vi "HFRR ADV v01.vi"() -> ()   [LabVIEW 2025] (continued)
        n1285 = local write "Zoom Factore"(100.0 ("Zoom Factore")) -> ()
        n1286 = Strip Path(path=w1421) -> (name=w1424:string)  [unwired: 1 out]
        n1287 = Match Pattern(string=w1424, regular expression=w1422) -> (match substring=w1423:string)  [unwired: 1 in, 3 out]
        n1288 = Equal?(x=w1423, y=w1422) -> (x = y?=w1420:bool)
        n1289 = case shown="False" w1420 {
          frame False {
            n1290 = local write "Magnification :"("10x" ("Magnification :")) -> ()
          }
          frame True {
            n1291 = local write "Magnification :"("5x" ("Magnification :")) -> ()
          }
        }
      }
    }
    n1292 = case shown="True" w1115 {
      selector: w1115 -> [_ w1403]
      tunnel: w1107 -> [w1400 w1408]
      tunnel: [w1400 w1402] -> _
      frame False {
      }
      frame True {
        n1293 = Not(x=w1403) -> (.not. x?=w1401:bool)
        n1294 = local read "Zoom Factore"() -> (w1406:dbl)
        n1295 = local write "OUT"(w1401) -> ()
        n1296 = call "IMAGE ANALYSIS.vi"("Enum"=POST_ANALYSIS_ENUM."ZOOM OUT", "error in"=w1408) -> ("error out"=w1402:errorcluster)  [unwired: 8 in, 1 out]
        n1297 = Divide(x=w1406, y=1.2) -> (x/y=w1404:dbl)
        n1298 = local write "Zoom Factore"(w1404) -> ()
      }
    }
    n1299 = case shown="True" w1116 {
      selector: w1116 -> [_ w1412]
      tunnel: w1107 -> [w1409 w1417]
      tunnel: [w1409 w1410] -> _
      frame False {
      }
      frame True {
        n1300 = Not(x=w1412) -> (.not. x?=w1411:bool)
        n1301 = local read "Zoom Factore"() -> (w1415:dbl)
        n1302 = local write "In"(w1411) -> ()
        n1303 = call "IMAGE ANALYSIS.vi"("Enum"=POST_ANALYSIS_ENUM."ZOOM IN", "error in"=w1417) -> ("error out"=w1410:errorcluster)  [unwired: 8 in, 1 out]
        n1304 = Multiply(x=w1415, y=1.2) -> (x*y=w1413:dbl)
        n1305 = local write "Zoom Factore"(w1413) -> ()
      }
    }
    n1306 = case shown="True" w1112 {
      selector: w1112 -> [_ w1384]
      tunnel: w1107 -> [w1382 w1386]
      tunnel: [w1382 w1385] -> _
      frame False {
      }
      frame True {
        n1307 = Not(x=w1384) -> (.not. x?=w1383:bool)
        n1308 = local write "Clear ROI Tool"(w1383) -> ()
        n1309 = call "IMAGE ANALYSIS.vi"("Enum"=POST_ANALYSIS_ENUM."CLEAR ROI", "error in"=w1386) -> ("error out"=w1385:errorcluster)  [unwired: 8 in, 1 out]
      }
    }
    n1310 = case shown="True" w1114 {
      selector: w1114 -> [_ w1396]
      tunnel: w1107 -> [w1394 w1399]
      tunnel: [w1394 w1397] -> _
      frame False {
      }
      frame True {
        n1311 = Not(x=w1396) -> (.not. x?=w1395:bool)
        n1312 = local write "line tool"(w1395) -> ()
        n1313 = call "IMAGE ANALYSIS.vi"("Enum"=POST_ANALYSIS_ENUM."DRAW LINE", "error in"=w1399) -> ("error out"=w1397:errorcluster)  [unwired: 8 in, 1 out]
      }
    }
    n1314 = case shown="True" w1113 {
      selector: w1113 -> [_ w1390]
      tunnel: w1107 -> [w1388 w1392]
      tunnel: [w1388 w1391] -> _
      frame False {
      }
      frame True {
        n1315 = Not(x=w1390) -> (.not. x?=w1389:bool)
        n1316 = local write "Rectangle Tool"(w1389) -> ()
        n1317 = call "IMAGE ANALYSIS.vi"("Enum"=POST_ANALYSIS_ENUM."DRAW REC", "error in"=w1392) -> ("error out"=w1391:errorcluster)  [unwired: 8 in, 1 out]
      }
    }
    n1318 = local read "SCAR MEASURMENT"() -> (w1100:enum32{"Auto Scar", "Manual Scar"})
    n1319 = local read "Fit to Screen Tool"() -> (w1109:bool)
    n1320 = local read "Resize Tool"() -> (w1108:bool)
    n1321 = case shown="\"Manual Scar\", Default" w1100 {
      frame "Auto Scar" {
        n1322 = property on="Cap Live Image" class="Bool (strict)"("BoolText.Text"="Report" ("Boolean Text.Text")) -> ()  [unwired: 2 in, 2 out]
      }
      frame "Manual Scar", Default {
        n1323 = property on="Cap Live Image" class="Bool (strict)"("BoolText.Text"="Save Image" ("Boolean Text.Text")) -> ()  [unwired: 2 in, 2 out]
      }
    }
    n1324 = local read "ROI Color Tool"() -> (w1110:bool)
    n1325 = local read "Pan Tool"() -> (w1111:bool)
    n1326 = case shown="True" w1111 {
      selector: w1111 -> [_ w1378]
      tunnel: w1107 -> [w1376 w1380]
      tunnel: [w1376 w1379] -> _
      frame False {
      }
      frame True {
        n1327 = Not(x=w1378) -> (.not. x?=w1377:bool)
        n1328 = call "IMAGE ANALYSIS.vi"("Enum"=POST_ANALYSIS_ENUM."PAN", "error in"=w1380) -> ("error out"=w1379:errorcluster)  [unwired: 8 in, 1 out]
        n1329 = local write "Pan Tool"(w1377) -> ()
      }
    }
    n1330 = case shown="True" w1108 {
      selector: w1108 -> [_ w1362]
      tunnel: w1107 -> [w1357 w1359]
      tunnel: [w1357 w1358] -> _
      frame False {
      }
      frame True {
        n1331 = Not(x=w1362) -> (.not. x?=w1361:bool)
        n1332 = local write "Resize Tool"(w1361) -> ()
        n1333 = call "IMAGE ANALYSIS.vi"("Enum"=POST_ANALYSIS_ENUM."RESIZE MODE", "error in"=w1359) -> ("error out"=w1358:errorcluster)  [unwired: 8 in, 1 out]
      }
    }
    n1334 = case shown="True" w1109 {
      selector: w1109 -> [_ w1367]
      tunnel: [w1363 w1368] -> _
      tunnel: w1107 -> [w1363 w1366]
      frame False {
      }
      frame True {
        n1335 = Not(x=w1367) -> (.not. x?=w1365:bool)
        n1336 = local write "Zoom Factore"(100.0 ("Zoom Factore")) -> ()
        n1337 = local write "Fit to Screen Tool"(w1365) -> ()
        n1338 = call "IMAGE ANALYSIS.vi"("Enum"=POST_ANALYSIS_ENUM."FIT", "error in"=w1366) -> ("error out"=w1368:errorcluster)  [unwired: 8 in, 1 out]
      }
    }
    n1339 = case shown="True" w1110 {
      selector: w1110 -> [_ w1373]
      tunnel: [w1370 w1374] -> _
      tunnel: w1107 -> [w1370 w1371]
      frame False {
      }
      frame True {
        n1340 = Not(x=w1373) -> (.not. x?=w1372:bool)
        n1341 = local write "ROI Color Tool"(w1372) -> ()
        n1342 = call "IMAGE ANALYSIS.vi"("Enum"=POST_ANALYSIS_ENUM."SET ROI COLOR", "error in"=w1371) -> ("error out"=w1374:errorcluster)  [unwired: 8 in, 1 out]
      }
    }
    n1343 = local read "Quit"() -> (w1124:bool)
  }
  n1344 = while {
    stop <- w1469 stop-if-true
    n1345 = local read "Image Path"() -> (w1472:path)
    n1346 = local read "Print 3"() -> (w1475:bool)
    n1347 = Equal?(x=w1472, y=path "") -> (x = y?=w1471:bool)
    n1348 = Not(x=w1471) -> (.not. x?=w1470:bool)
    n1349 = property on="Print 3" class="Bool (strict)"("Visible"=w1470) -> ()  [unwired: 2 in, 2 out]
    n1350 = case shown="True" w1475 {
      frame False {
        n1351 = local write "Rd"(TRUE ("Boolean 7")) -> ()
      }
      frame True {
        n1352 = flat-sequence {
          tunnel: [w1515] -> w1483
          tunnel: [w1502] -> w1481
          tunnel: [w1512] -> w1477
          tunnel: w1483 -> [w1524]
          tunnel: [w1524] -> w1482
          tunnel: w1481 -> [w1523]
          tunnel: [w1523] -> w1480
          tunnel: [w1521] -> w1479
          tunnel: [w1520] -> w1478
          tunnel: w1477 -> [w1520]
          tunnel: w1482 -> [w1526]
          tunnel: w1480 -> [w1527]
          tunnel: w1479 -> [_]
          tunnel: w1478 -> [w1525]
          frame #0 {
            n1353 = case shown="True" "Rd" {
              frame False {
              }
              frame True {
                n1354 = while {
                  tunnel: "abcdefABCDEF" ("string 2") -> [w1494]
                  shift-right: [w1492] -> w1486
                  shift-left: "" -> [w1491]
                  i -> [w1501]
                  stop <- w1500 stop-if-true
                  n1355 = Random Number (0-1)() -> (number: 0 to 1=w1495:dbl)
                  n1356 = Multiply(x=w1495, y=62.0) -> (x*y=w1497:dbl)
                  n1357 = Decrement(x="Length 2") -> (x-1=w1490:i16)
                  n1358 = To Word Integer(number=w1497) -> (16bit integer=w1498:i16)
                  n1359 = String Subset(string=w1494, offset (0)=w1498, length (rest)=1 ("length (rest)")) -> (substring=w1493:string)
                  n1360 = Greater Or Equal?(x=w1501, y=w1490) -> (x >= y?=w1500:bool)
                  n1361 = Concatenate Strings(w1493, w1491) -> (w1492:string)
                }
                "String 10" <- w1486
                n1362 = local write "Rd"(FALSE ("Boolean 7")) -> ()
              }
            }
          }
          frame #1 {
            w1513 = "_resized.jpg" ("command line")
            (unwired) ".jpg -resize 320x240 " ("string")
            (unwired) "Choose an Image File" ("prompt")
            # "-resize 1798x425"
            n1363 = local read "Image Path"() -> (w1507:path)
            n1364 = Strip Path(path=w1507) -> (stripped path=w1502:path, name=w1503:string)
            n1365 = Match Pattern(string=w1503, regular expression=".jpg") -> (before substring=→"before substring 2":string, after substring=→"after substring":string)  [unwired: 1 in, 2 out]
            n1366 = Match Pattern(string=w1503, regular expression="\\") -> (before substring=w1509:string)  [unwired: 1 in, 3 out]
            n1367 = Match Pattern(string=w1509, regular expression=".jpg") -> (before substring=w1508:string)  [unwired: 1 in, 3 out]
            n1368 = Concatenate Strings("cmd /c convert " ("string"), w1508, ".jpg -resize 320x240  " ("command line"), w1508, w1513) -> (w1516:string)
            n1369 = call <vilib>:"System Exec.vi"("run minimized? (F)"=TRUE, "wait until completion? (T)"=TRUE, "working directory"=w1502, "command line"=w1516) -> ("error out"=w1515:errorcluster)  [unwired: 4 in, 3 out]
            "error out 2" <- w1515
            n1370 = Concatenate Strings(w1508, w1513) -> (w1512:string)
          }
          frame #2 {
            n1371 = Wait (ms)(milliseconds to wait=u32 2000 ("millisecond timer value")) -> (millisecond timer value=w1521:u32)
          }
          frame #3 {
            n1372 = case shown="No Error" w1526 {
              tunnel: w1527 -> [w1530 _]
              tunnel: w1525 -> [w1528 _]
              frame No Error {
                (unwired) ".jpg" ("string")
                n1373 = Path To String(path=w1530) -> (string=w1534:string)
                n1374 = Concatenate Strings(w1534, "\\" ("string"), w1528) -> (w1533:string)
                n1375 = String To Path(string=w1533) -> (path=w1532:path)
                n1376 = call <vilib>:"Read JPEG File.vi"("path to JPEG file"=w1532) -> ("image data"=w1536:T2)  [unwired: 8 in, 2 out]
                "image data" <- w1536
                n1377 = local write "Print 3"(FALSE ("Print 2")) -> ()
                n1378 = call <vilib>:"Draw Flattened Pixmap.vi"("image data"=w1536) -> ("new picture"=→"new picture":picture)  [unwired: 8 in]
              }
              frame Error {
              }
            }
          }
        }
      }
    }
    n1379 = Wait (ms)(milliseconds to wait=u32 20 ("millisecond timer value")) -> ()  [unwired: 1 out]
    n1380 = local read "Quit"() -> (w1469:bool)
  }
  n1381 = while {
    tunnel: w44 -> [_]
    tunnel: w30 -> [_]
    stop <- w1565 stop-if-true
    # "New Adv Logics"
    n1382 = local read "Main Tab"() -> (w1548:T4)
    n1383 = local read "Sign In"() -> (w1563:bool)
    n1384 = case shown="\"Advance\"" w1548 {
      frame "HOME", Default {
        n1385 = local read "LIVE FEED MIN TEMP"() -> (w1713:bool)
        n1386 = local write "LIVE FEED MAX TEMP"(TRUE ("LIVE FEED MAX TEMP")) -> ()
        n1387 = local read "CAMERA ROI MIN TEMP"() -> (w1711:bool)
        n1388 = case shown="True" w1713 {
          selector: w1713 -> [_ w1720]
          frame False {
          }
          frame True {
            n1389 = Not(x=w1720) -> (.not. x?=w1719:bool)
            n1390 = local write "LIVE FEED MIN TEMP"(w1719) -> ()
            n1391 = call "CAMERA LIVE FEED FGV.vi"("Enum - Menu"=CAMERA_LIVE_FEED_ENUM."CAMERA MINIMIZE") -> ()  [unwired: 9 in, 2 out]
          }
        }
        n1392 = case shown="True" w1711 {
          selector: w1711 -> [_ w1717]
          frame False {
          }
          frame True {
            n1393 = Not(x=w1717) -> (.not. x?=w1716:bool)
            n1394 = local write "CAMERA ROI MIN TEMP"(w1716) -> ()
            n1395 = call "IMAGE ANALYSIS.vi"("Enum"=POST_ANALYSIS_ENUM."MINIMIZE UI") -> ()  [unwired: 9 in, 2 out]
          }
        }
        n1396 = local write "CAMERA ROI MAX TEMP"(TRUE ("CAMERA ROI MAX TEMP")) -> ()
      }
      frame "Test Setup" {
        n1397 = local read "LIVE FEED MIN TEMP"() -> (w1723:bool)
        n1398 = local read "CAMERA ROI MIN TEMP"() -> (w1721:bool)
        n1399 = local write "LIVE FEED MAX TEMP"(TRUE ("LIVE FEED MAX TEMP")) -> ()
        n1400 = case shown="True" w1723 {
          selector: w1723 -> [_ w1730]
          frame False {
          }
          frame True {
            n1401 = Not(x=w1730) -> (.not. x?=w1729:bool)
            n1402 = local write "LIVE FEED MIN TEMP"(w1729) -> ()
            n1403 = call "CAMERA LIVE FEED FGV.vi"("Enum - Menu"=CAMERA_LIVE_FEED_ENUM."CAMERA MINIMIZE") -> ()  [unwired: 9 in, 2 out]
          }
        }
        n1404 = case shown="True" w1721 {
          selector: w1721 -> [_ w1727]
          frame False {
          }
          frame True {
            n1405 = Not(x=w1727) -> (.not. x?=w1726:bool)
            n1406 = local write "CAMERA ROI MIN TEMP"(w1726) -> ()
            n1407 = call "IMAGE ANALYSIS.vi"("Enum"=POST_ANALYSIS_ENUM."MINIMIZE UI") -> ()  [unwired: 9 in, 2 out]
          }
        }
        n1408 = local write "CAMERA ROI MAX TEMP"(TRUE ("CAMERA ROI MAX TEMP")) -> ()
      }
      frame "Acquire" {
        n1409 = local read "LIVE FEED MIN TEMP"() -> (w1733:bool)
        n1410 = local write "LIVE FEED MAX TEMP"(TRUE ("LIVE FEED MAX TEMP")) -> ()
        n1411 = local read "CAMERA ROI MIN TEMP"() -> (w1731:bool)
        n1412 = case shown="True" w1733 {
          selector: w1733 -> [_ w1740]
          frame False {
          }
          frame True {
            n1413 = Not(x=w1740) -> (.not. x?=w1739:bool)
            n1414 = local write "LIVE FEED MIN TEMP"(w1739) -> ()
            n1415 = call "CAMERA LIVE FEED FGV.vi"("Enum - Menu"=CAMERA_LIVE_FEED_ENUM."CAMERA MINIMIZE") -> ()  [unwired: 9 in, 2 out]
          }
        }
        n1416 = case shown="True" w1731 {
          selector: w1731 -> [_ w1737]
          frame False {
          }
          frame True {
            n1417 = Not(x=w1737) -> (.not. x?=w1736:bool)
            n1418 = local write "CAMERA ROI MIN TEMP"(w1736) -> ()
            n1419 = call "IMAGE ANALYSIS.vi"("Enum"=POST_ANALYSIS_ENUM."MINIMIZE UI") -> ()  [unwired: 9 in, 2 out]
          }
        }
        n1420 = local write "CAMERA ROI MAX TEMP"(TRUE ("CAMERA ROI MAX TEMP")) -> ()
      }
      frame "Adv Scar" {
        n1421 = local read "CAMERA ROI MIN TEMP"() -> (w1741:bool)
        n1422 = case shown="True" "LIVE FEED MAX TEMP" {
          selector: "LIVE FEED MAX TEMP" -> [_ w1762]
          frame False {
          }
          frame True {
            n1423 = Not(x=w1762) -> (.not. x?=w1761:bool)
            n1424 = local write "LIVE FEED MAX TEMP"(w1761) -> ()
            n1425 = call "CAMERA LIVE FEED FGV.vi"("Enum - Menu"=CAMERA_LIVE_FEED_ENUM."CAMERA RESTORE") -> ("error out"=w1752:errorcluster)  [unwired: 9 in, 1 out]
            n1426 = Type Cast(type=30, x=0) -> (*(type *) &x=w1756:i32)
            n1427 = Add(x=w1756, y=48) -> (x+y=w1757:i32)
            n1428 = call "CAMERA LIVE FEED FGV.vi"("Enum - Menu"=CAMERA_LIVE_FEED_ENUM."CAMERA MODE SET", "error in (no error)"=w1752, "CAMERA MODE"=w1757) -> ("error out"=w1749:errorcluster)  [unwired: 7 in, 1 out]
            n1429 = call "CAMERA LIVE FEED FGV.vi"("Enum - Menu"=CAMERA_LIVE_FEED_ENUM."CAMERA GRAY", "error in (no error)"=w1749) -> ("error out"=w1748:errorcluster)  [unwired: 8 in, 1 out]
            n1430 = call "LIST FILE NAMES.vi"("error in (no error)"=w1748) -> ("error out"=w1758:errorcluster, "filenames"=w1759:string[])  [unwired: 9 in]
            n1431 = property on="FILE 3" class="CmbBox"(error in=w1758, "Strings[]"=w1759) -> ()  [unwired: 1 in, 2 out]
          }
        }
        n1432 = case shown="True" w1741 {
          selector: w1741 -> [_ w1747]
          frame False {
          }
          frame True {
            n1433 = Not(x=w1747) -> (.not. x?=w1746:bool)
            n1434 = local write "CAMERA ROI MIN TEMP"(w1746) -> ()
            n1435 = call "IMAGE ANALYSIS.vi"("Enum"=POST_ANALYSIS_ENUM."MINIMIZE UI") -> ()  [unwired: 9 in, 2 out]
          }
        }
        n1436 = local write "CAMERA ROI MAX TEMP"(TRUE ("CAMERA ROI MAX TEMP")) -> ()
        "LIVE FEED MIN TEMP" <- TRUE ("LIVE FEED MIN TEMP")
      }
      frame "Adv Scar Report" {
        n1437 = local read "CAMERA ROI MAX TEMP"() -> (w1763:bool)
        n1438 = local read "LIVE FEED MIN TEMP"() -> (w1765:bool)
        n1439 = local write "LIVE FEED MAX TEMP"(TRUE ("LIVE FEED MAX TEMP")) -> ()
        n1440 = case shown="True" w1765 {
          selector: w1765 -> [_ w1774]
          frame False {
          }
          frame True {
            n1441 = Not(x=w1774) -> (.not. x?=w1773:bool)
            n1442 = local write "LIVE FEED MIN TEMP"(w1773) -> ()
            n1443 = call "CAMERA LIVE FEED FGV.vi"("Enum - Menu"=CAMERA_LIVE_FEED_ENUM."CAMERA MINIMIZE") -> ()  [unwired: 9 in, 2 out]
          }
        }
        n1444 = case shown="True" w1763 {
          selector: w1763 -> [_ w1771]
          frame False {
          }
          frame True {
            n1445 = Not(x=w1771) -> (.not. x?=w1769:bool)
            n1446 = local write "CAMERA ROI MAX TEMP"(w1769) -> ()
            n1447 = call "IMAGE ANALYSIS.vi"("Enum"=POST_ANALYSIS_ENUM."SHOW UI") -> ("error out"=w1768:errorcluster)  [unwired: 9 in, 1 out]
            n1448 = call "LIST FILE NAMES.vi"("error in (no error)"=w1768) -> ("filenames"=w1767:string[])  [unwired: 9 in, 1 out]
            n1449 = property on="Test File List :" class="CmbBox"("Strings[]"=w1767) -> ()  [unwired: 2 in, 2 out]
          }
        }
        n1450 = local write "CAMERA ROI MIN TEMP"(TRUE ("CAMERA ROI MIN TEMP")) -> ()
      }
      frame "Compare Files" {
        n1451 = local read "LIVE FEED MIN TEMP"() -> (w1777:bool)
        n1452 = local write "LIVE FEED MAX TEMP"(TRUE ("LIVE FEED MAX TEMP")) -> ()
        n1453 = local read "CAMERA ROI MIN TEMP"() -> (w1775:bool)
        n1454 = case shown="True" w1777 {
          selector: w1777 -> [_ w1784]
          frame False {
          }
          frame True {
            n1455 = Not(x=w1784) -> (.not. x?=w1783:bool)
            n1456 = local write "LIVE FEED MIN TEMP"(w1783) -> ()
            n1457 = call "CAMERA LIVE FEED FGV.vi"("Enum - Menu"=CAMERA_LIVE_FEED_ENUM."CAMERA MINIMIZE") -> ()  [unwired: 9 in, 2 out]
          }
        }
        n1458 = case shown="True" w1775 {
          selector: w1775 -> [_ w1781]
          frame False {
          }
          frame True {
            n1459 = Not(x=w1781) -> (.not. x?=w1780:bool)
            n1460 = local write "CAMERA ROI MIN TEMP"(w1780) -> ()
            n1461 = call "IMAGE ANALYSIS.vi"("Enum"=POST_ANALYSIS_ENUM."MINIMIZE UI") -> ()  [unwired: 9 in, 2 out]
          }
        }
        n1462 = local write "CAMERA ROI MAX TEMP"(TRUE ("CAMERA ROI MAX TEMP")) -> ()
      }
      frame "About" {
        n1463 = local read "LIVE FEED MIN TEMP"() -> (w1787:bool)
        n1464 = local write "LIVE FEED MAX TEMP"(TRUE ("LIVE FEED MAX TEMP")) -> ()
        n1465 = local read "CAMERA ROI MIN TEMP"() -> (w1786:bool)
        n1466 = case shown="True" w1787 {
          selector: w1787 -> [_ w1794]
          frame False {
          }
          frame True {
            n1467 = Not(x=w1794) -> (.not. x?=w1793:bool)
            n1468 = local write "LIVE FEED MIN TEMP"(w1793) -> ()
            n1469 = call "CAMERA LIVE FEED FGV.vi"("Enum - Menu"=CAMERA_LIVE_FEED_ENUM."CAMERA MINIMIZE") -> ()  [unwired: 9 in, 2 out]
          }
        }
        n1470 = case shown="True" w1786 {
          selector: w1786 -> [_ w1791]
          frame False {
          }
          frame True {
            n1471 = Not(x=w1791) -> (.not. x?=w1790:bool)
            n1472 = local write "CAMERA ROI MIN TEMP"(w1790) -> ()
            n1473 = call "IMAGE ANALYSIS.vi"("Enum"=POST_ANALYSIS_ENUM."MINIMIZE UI") -> ()  [unwired: 9 in, 2 out]
          }
        }
        n1474 = local write "CAMERA ROI MAX TEMP"(TRUE ("CAMERA ROI MIN TEMP")) -> ()
      }
      frame "Advance" {
        n1475 = local read "LIVE FEED MIN TEMP"() -> (w1797:bool)
        n1476 = local write "LIVE FEED MAX TEMP"(TRUE ("LIVE FEED MAX TEMP")) -> ()
        n1477 = local read "CAMERA ROI MIN TEMP"() -> (w1795:bool)
        n1478 = case shown="True" w1797 {
          selector: w1797 -> [_ w1804]
          frame False {
          }
          frame True {
            n1479 = Not(x=w1804) -> (.not. x?=w1803:bool)
            n1480 = local write "LIVE FEED MIN TEMP"(w1803) -> ()
            n1481 = call "CAMERA LIVE FEED FGV.vi"("Enum - Menu"=CAMERA_LIVE_FEED_ENUM."CAMERA MINIMIZE") -> ()  [unwired: 9 in, 2 out]
          }
        }
        n1482 = local write "CAMERA ROI MAX TEMP"(TRUE ("CAMERA ROI MAX TEMP")) -> ()
        n1483 = case shown="True" w1795 {
          selector: w1795 -> [_ w1801]
          frame False {
          }
          frame True {
            n1484 = Not(x=w1801) -> (.not. x?=w1800:bool)
            n1485 = local write "CAMERA ROI MIN TEMP"(w1800) -> ()
            n1486 = call "IMAGE ANALYSIS.vi"("Enum"=POST_ANALYSIS_ENUM."MINIMIZE UI") -> ()  [unwired: 9 in, 2 out]
          }
        }
      }
      frame "Mooha" {
        n1487 = local read "LIVE FEED MIN TEMP"() -> (w1807:bool)
        n1488 = local write "LIVE FEED MAX TEMP"(TRUE ("LIVE FEED MAX TEMP")) -> ()
        n1489 = local read "CAMERA ROI MIN TEMP"() -> (w1805:bool)
        n1490 = case shown="True" w1807 {
          selector: w1807 -> [_ w1814]
          frame False {
          }
          frame True {
            n1491 = Not(x=w1814) -> (.not. x?=w1813:bool)
            n1492 = local write "LIVE FEED MIN TEMP"(w1813) -> ()
            n1493 = call "CAMERA LIVE FEED FGV.vi"("Enum - Menu"=CAMERA_LIVE_FEED_ENUM."CAMERA MINIMIZE") -> ()  [unwired: 9 in, 2 out]
          }
        }
        n1494 = local write "CAMERA ROI MAX TEMP"(TRUE ("CAMERA ROI MAX TEMP")) -> ()
        n1495 = case shown="True" w1805 {
          selector: w1805 -> [_ w1811]
          frame False {
          }
          frame True {
            n1496 = Not(x=w1811) -> (.not. x?=w1810:bool)
            n1497 = local write "CAMERA ROI MIN TEMP"(w1810) -> ()
            n1498 = call "IMAGE ANALYSIS.vi"("Enum"=POST_ANALYSIS_ENUM."MINIMIZE UI") -> ()  [unwired: 9 in, 2 out]
          }
        }
      }
    }
    n1499 = property on="DEMO" class="Bool (strict)"() -> ("Value"=w1537:bool)  [unwired: 2 in, 2 out]
    n1500 = local read "Auto Start Test"() -> (w1540:bool)
    n1501 = case shown="False" w1537 {
      frame False {
        n1502 = local read "Main Tab"() -> (w1566:T4)
        n1503 = case shown="\"HOME\"" w1566 {
          frame "HOME" {
            n1504 = local write "main tab sub"(enum32{"Page 1", "Page 2"}."Page 1" ("main tab sub")) -> ()
          }
          frame Default {
            n1505 = local write "main tab sub"(enum32{"Page 1", "Page 2"}."Page 2" ("main tab sub")) -> ()
          }
        }
      }
      frame True {
      }
    }
    n1506 = case shown="True" "sign in temp" {
      frame False {
      }
      frame True {
        w1651 = 1 ("y")
        n1507 = local read "USERNAME"() -> (w1657:string)
        n1508 = local read "USER ID"() -> (w1654:string)
        n1509 = call <vilib>:"Trim Whitespace.vi"("string"=w1657) -> ("trimmed string"=w1656:string)  [unwired: 1 in]
        n1510 = call <vilib>:"Trim Whitespace.vi"("string"=w1654) -> ("trimmed string"=w1655:string)  [unwired: 1 in]
        n1511 = String Length(string=w1656) -> (length=w1653:i32)
        n1512 = String Length(string=w1655) -> (length=w1652:i32)
        n1513 = Greater?(x=w1653, y=w1651) -> (0:w1650:bool)
        n1514 = Greater?(x=w1652, y=w1651) -> (0:w1649:bool)
        n1515 = And(x=w1650, y=w1649) -> (x .and. y?=w1648:bool)
        n1516 = case shown="True" w1648 {
          frame False {
            n1517 = property on="Sign In" class="Bool (strict)"("DisabledEnum"=T20."Disabled" ("Disabled")) -> ()  [unwired: 2 in, 2 out]
          }
          frame True {
            n1518 = property on="Sign In" class="Bool (strict)"("DisabledEnum"=T20."Enabled" ("Disabled")) -> ()  [unwired: 2 in, 2 out]
          }
        }
      }
    }
    n1519 = local read "Air Temperature"() -> (w1556:bool)
    n1520 = property on="DEMO" class="Bool (strict)"() -> ("Value"=w1538:bool)  [unwired: 2 in, 2 out]
    n1521 = local read "Coefficient Of Friction"() -> (w1557:bool)
    n1522 = case shown="False" w1540 {
      frame False {
        n1523 = local read "Auto stop temp"() -> (w1645:bool)
        n1524 = case shown="True" w1645 {
          frame False {
          }
          frame True {
            n1525 = local write "Auto Start Temp"(FALSE ("Auto Start Temp")) -> ()
          }
        }
      }
      frame True {
        "Auto stop temp" <- TRUE ("Auto stop temp")
      }
    }
    n1526 = local read "Humidity 3"() -> (w1555:bool)
    n1527 = case shown="True" w1563 {
      selector: w1563 -> [_ w1920]
      frame False {
      }
      frame True {
        n1528 = Not(x=w1920) -> (.not. x?=w1919:bool)
        n1529 = local write "Sign In"(w1919) -> ()
        n1530 = local write "Main Dashboard Buttons"(T26."Test Setup" ("Main Dashboard Buttons")) -> ()
      }
    }
    n1531 = case shown="\"Numeric Display\", Default" "Num/Graph" {
      frame "Numeric Display", Default {
        n1532 = property on="Single/Multiple" class="RadioBtnsControl (strict)"("Visible"=FALSE) -> ()  [unwired: 2 in, 2 out]
        n1533 = property on="Single - Graph" class="Ring (strict)"("Visible"=FALSE) -> ()  [unwired: 2 in, 2 out]
        n1534 = local write "Main Tab Display"(T6."Dashboard 1" ("Main Tab Display")) -> ()
      }
      frame "Graph Display" {
        n1535 = property on="Single/Multiple" class="RadioBtnsControl (strict)"("Visible"=TRUE) -> ()  [unwired: 2 in, 2 out]
        n1536 = case shown="\"Multiple\"" "Single/Multiple" {
          frame "Single ", Default {
            n1537 = property on="Single - Graph" class="Ring (strict)"("Visible"=TRUE) -> ()  [unwired: 2 in, 2 out]
            n1538 = local write "Main Tab Display"(T6."Dashboard 3" ("Main Tab Display")) -> ()
          }
          frame "Multiple" {
            n1539 = property on="Single - Graph" class="Ring (strict)"("Visible"=FALSE) -> ()  [unwired: 2 in, 2 out]
            n1540 = local write "Main Tab Display"(T6."Dashboard 2" ("Main Tab Display")) -> ()
          }
        }
      }
    }
    n1541 = local read "Stroke"() -> (w1554:bool)
    n1542 = local read "USERNAME"() -> (w1559:string)
    n1543 = case shown="False" w1538 {
      frame False {
        n1544 = case shown="\"Calibration\"" "Main Dashboard Buttons" {
          tunnel: [T4."HOME" ("Main Tab") T4."Test Setup" ("Main Tab") T4."Acquire" ("Main Tab") T4."Adv Scar" ("Main Tab") T4."Adv Scar Report" ("Main Tab") T4."Compare Files" ("Main Tab") T4."Calibration" ("Main Tab") T4."About" ("Main Tab") T4."Advance" ("Main Tab")] -> w1569
          frame "Home", Default {
          }
          frame "Test Setup" {
          }
          frame "Dashboard" {
          }
          frame "Imaging" {
          }
          frame "Report" {
          }
          frame "Analysis" {
          }
          frame "Calibration" {
          }
          frame "About" {
          }
          frame "Advance" {
          }
        }
        n1545 = local write "Main Tab"(w1569) -> ()
      }
      frame True {
      }
    }
    n1546 = case shown="True" w1557 {
      selector: w1557 -> [_ w1854]
      frame False {
      }
      frame True {
        n1547 = Not(x=w1854) -> (.not. x?=w1853:bool)
        n1548 = local write "Coefficient Of Friction"(w1853) -> ()
        n1549 = local write "Tab Control 2"(T8."Coefficient Of Friction" ("Tab Control 2")) -> ()
      }
    }
    n1550 = case shown="True" w1556 {
      selector: w1556 -> [_ w1851]
      frame False {
      }
      frame True {
        n1551 = Not(x=w1851) -> (.not. x?=w1849:bool)
        n1552 = local write "Air Temperature"(w1849) -> ()
        n1553 = local write "Tab Control 2"(T8."Air Temperature" ("Tab Control 2")) -> ()
      }
    }
    n1554 = case shown="True" w1554 {
      selector: w1554 -> [_ w1845]
      frame False {
      }
      frame True {
        n1555 = Not(x=w1845) -> (.not. x?=w1843:bool)
        n1556 = local write "Stroke"(w1843) -> ()
        n1557 = local write "Tab Control 2"(T8."Stroke" ("Tab Control 2")) -> ()
      }
    }
    n1558 = local write "tested by"(w1559) -> ()
    n1559 = case shown="True" w1555 {
      selector: w1555 -> [_ w1848]
      frame False {
      }
      frame True {
        n1560 = Not(x=w1848) -> (.not. x?=w1846:bool)
        n1561 = local write "Humidity 3"(w1846) -> ()
        n1562 = local write "Tab Control 2"(T8."Humidity" ("Tab Control 2")) -> ()
      }
    }
    n1563 = Wait (ms)(milliseconds to wait=u32 100) -> ()  [unwired: 1 out]
    n1564 = local read "Main Tab Display"() -> (w1558:T6)
    n1565 = case shown="\"Dashboard 3\"" w1558 {
      frame "Dashboard 1", Default {
        n1566 = property on="Reset Graph" class="Bool (strict)"("Visible"=FALSE) -> ()  [unwired: 2 in, 2 out]
      }
      frame "Dashboard 2" {
        n1567 = property on="Reset Graph" class="Bool (strict)"("Visible"=TRUE) -> ()  [unwired: 2 in, 2 out]
      }
      frame "Dashboard 3" {
        n1568 = property on="Reset Graph" class="Bool (strict)"("Visible"=TRUE) -> ()  [unwired: 2 in, 2 out]
      }
    }
    n1569 = local read "SCAR MEASURMENT"() -> (w1546:enum32{"Auto Scar", "Manual Scar"})
    n1570 = local read "Humidity"() -> (w1560:bool)
    n1571 = local read "Cap Live Image"() -> (w1543:bool)
    n1572 = local read "Sample Temperature"() -> (w1553:bool)
    n1573 = local read "Air Temp vs Humidity"() -> (w1551:bool)
    n1574 = local read "Frequency"() -> (w1552:bool)
    n1575 = case shown="False" w1560 {
      frame False {
        n1576 = local write "Humidity On Command"(TRUE ("Humidity On Command")) -> ()
        n1577 = case shown="True" "Humidity Off Command" {
          selector: "Humidity Off Command" -> [_ w1861]
          frame False {
          }
          frame True {
            n1578 = stacked-sequence {
              frame #0 {
                n1579 = local read "WriteHumidity"() -> (w1863:string[])
                n1580 = Insert Into Array(array=w1863, new element="R;1" ("new element/subarray")) -> (w1862:string[])  [unwired: 1 in]
                n1581 = local write "WriteHumidity"(w1862) -> ()
              }
              frame #1 {
                n1582 = Wait (ms)(milliseconds to wait=u32 500) -> ()  [unwired: 1 out]
              }
              frame #2 {
                n1583 = local read "WriteHumidity"() -> (w1867:string[])
                n1584 = local read "EVENT LOG"() -> (w1871:string)
                n1585 = call "Event Log.vi"("Content"="Humidity Control Off" ("string"), "EVENT LOG"=w1871) -> ("EVENT LOG"=w1872:string)  [unwired: 8 in, 1 out]
                n1586 = local write "EVENT LOG"(w1872) -> ()
                n1587 = Insert Into Array(array=w1867, new element="R;1" ("new element/subarray")) -> (w1868:string[])  [unwired: 1 in]
                n1588 = local write "WriteHumidity"(w1868) -> ()
                n1589 = local write "Humidity 2"(TRUE ("Humidity")) -> ()
              }
            }
            n1590 = Not(x=w1861) -> (.not. x?=w1860:bool)
            n1591 = local write "Humidity Off Command"(w1860) -> ()
          }
        }
      }
      frame True {
        n1592 = local write "Humidity Off Command"(TRUE ("Humidity Off Command")) -> ()
        n1593 = case shown="False" "Humidity On Command" {
          selector: "Humidity On Command" -> [_ w1876]
          frame False {
          }
          frame True {
            n1594 = stacked-sequence {
              frame #0 {
                n1595 = local read "Set Rh"() -> (w1882:dbl)
                n1596 = local read "WriteHumidity"() -> (w1878:string[])
                n1597 = Number To Fractional String(number=w1882, precision (6)=i16 2) -> (F-format string=w1883:string)  [unwired: 2 in]
                n1598 = Concatenate Strings("M;" ("new element/subarray"), w1883) -> (w1881:string)
                n1599 = Insert Into Array(array=w1878, new element=w1881) -> (w1877:string[])  [unwired: 1 in]
                n1600 = local write "WriteHumidity"(w1877) -> ()
              }
              frame #1 {
                n1601 = Wait (ms)(milliseconds to wait=u32 500) -> ()  [unwired: 1 out]
              }
              frame #2 {
                n1602 = local read "WriteHumidity"() -> (w1886:string[])
                n1603 = local read "Set Rh"() -> (w1890:dbl)
                n1604 = Number To Fractional String(number=w1890, precision (6)=i16 2) -> (F-format string=w1891:string)  [unwired: 2 in]
                n1605 = Concatenate Strings("M;" ("new element/subarray"), w1891) -> (w1889:string)
                n1606 = Insert Into Array(array=w1886, new element=w1889) -> (w1885:string[])  [unwired: 1 in]
                n1607 = local write "WriteHumidity"(w1885) -> ()
              }
              frame #3 {
                n1608 = Wait (ms)(milliseconds to wait=u32 500) -> ()  [unwired: 1 out]
              }
              frame #4 {
                (unwired) "% RH" ("string")
                (unwired) i16 2 ("precision (6)")
                (unwired) "M;" ("new element/subarray")
                n1609 = local read "Set Rh"() -> (w1900:dbl)
                n1610 = local read "WriteHumidity"() -> (w1893:string[])
                n1611 = Number To Fractional String(number=w1900, precision (6)=i16 2) -> (F-format string=w1897:string)  [unwired: 2 in]
                n1612 = Concatenate Strings("M;" ("new element/subarray"), w1897) -> (w1901:string)
                n1613 = Concatenate Strings("Humidity Set to : " ("string"), w1897, "% RH" ("string")) -> (w1895:string)
                n1614 = Insert Into Array(array=w1893, new element=w1901) -> (w1894:string[])  [unwired: 1 in]
                n1615 = disable-structure shown="Enabled" {
                  frame Enabled {
                    n1616 = local read "EVENT LOG"() -> (w1904:string)
                    n1617 = call "Event Log.vi"("Content"="Humidity Control On", "EVENT LOG"=w1904) -> ("EVENT LOG"=w1905:string)  [unwired: 8 in, 1 out]
                    n1618 = local write "EVENT LOG"(w1905) -> ()
                  }
                  frame Disabled {
                  }
                }
                n1619 = disable-structure shown="Enabled" {
                  disable-tunnel: w1895 -> [_ _]
                  frame Enabled {
                    n1620 = local read "EVENT LOG"() -> (w1907:string)
                    n1621 = call "Event Log.vi"("Content"="Humidity Control On", "EVENT LOG"=w1907) -> ("EVENT LOG"=w1908:string)  [unwired: 8 in, 1 out]
                    n1622 = local write "EVENT LOG"(w1908) -> ()
                  }
                  frame Disabled {
                  }
                }
                n1623 = local write "WriteHumidity"(w1894) -> ()
              }
            }
            n1624 = Not(x=w1876) -> (.not. x?=w1875:bool)
            n1625 = local write "Humidity On Command"(w1875) -> ()
          }
        }
      }
    }
    n1626 = Equal?(x=w1546, y=enum32{"Auto Scar", "Manual Scar"}."Auto Scar" ("SCAR MEASURMENT")) -> (x = y?=w1542:bool)
    n1627 = local read "TEST STANDARD"() -> (w1549:T5)
    n1628 = And(x=w1543, y=w1542) -> (x .and. y?=w1544:bool)
    n1629 = case shown="True" w1544 {
      selector: w1544 -> [_ w1660]
      tunnel: errorcluster {"status"=FALSE, "code"=0, "source"=""} ("error in (no error) 3") -> [_ w1661]
      frame False {
      }
      frame True {
        n1630 = stacked-sequence {
          tunnel: w1661 -> [_ _ _ _ _ _ _ w1709]
          tunnel: w1660 -> [_ _ _ _ _ w1690 _ _]
          frame #0 {
            n1631 = call "CAMERA LIVE FEED FGV.vi"("Enum - Menu"=CAMERA_LIVE_FEED_ENUM."CAMERA MINIMIZE") -> ()  [unwired: 9 in, 2 out]
          }
          frame #1 {
            n1632 = property on="Auto Scar Check  2" class="Clust (strict)"("Visible"=TRUE) -> ()  [unwired: 2 in, 2 out]
          }
          frame #2 {
            n1633 = String To Path(string="C:\\LAB-IQ\\Image Calibrate v01.dcf") -> (path=w1666:path)
            n1634 = Open/Create/Replace File ("Open File")(file path (use dialog)=w1666) -> (refnum out=w1667:refnum<file>)  [unwired: 5 in, 2 out]
            n1635 = for {
              N: 4 -> [_]
              tunnel: w1667 -> [w1673]
              i -> [w1669]
              n1636 = Read from Text File ("Read File")(file (use dialog)=w1673) -> (text=w1674:string)  [unwired: 3 in, 3 out]
              n1637 = String Subset(string=w1674, offset (0)=6, length (rest)=10 ("length (rest)")) -> (substring=w1670:string)
              n1638 = Fract/Exp String To Number(string=w1670) -> (number=w1668:dbl)  [unwired: 3 in, 1 out]
              n1639 = case shown="0" w1669 {
                tunnel: w1668 -> [w1675 w1676 _ w1677 _]
                frame 0 {
                  "5x Gain" <- w1675
                }
                frame 1 {
                  "10x Gain" <- w1676
                }
                frame 2 {
                }
                frame 3 {
                  "100x gain" <- w1677
                }
                frame 4, Default {
                }
              }
            }
          }
          frame #3 {
            n1640 = local read "FILE 3"() -> (w1683:string)
            n1641 = call <vilib>:"Trim Whitespace.vi"("string"="C:\\LAB-IQ\\images\\") -> ("trimmed string"=w1685:string)  [unwired: 1 in]
            n1642 = String To Path(string=w1685) -> (path=w1684:path)
            n1643 = Concatenate Strings(w1683, ".png" ("string")) -> (w1682:string)
            n1644 = Build Path(base path=w1684, name or relative path=w1682) -> (appended path=w1680:path)
            "Image path" <- w1680
            n1645 = Path To String(path=w1680) -> (string=w1679:string)
            n1646 = call "CAMERA LIVE FEED FGV.vi"("Enum - Menu"=CAMERA_LIVE_FEED_ENUM."CAMERA SAVE", "Image Path"=w1679) -> ()  [unwired: 8 in, 2 out]
          }
          frame #4 {
            n1647 = One Button Dialog(message="Image saved successfully") -> ()  [unwired: 1 in, 1 out]
          }
          frame #5 {
            n1648 = local read "TEST STANDARD"() -> (w1689:T5)
            n1649 = local read "Magnification len live scar"() -> (w1701:string)
            n1650 = Not(x=w1690) -> (.not. x?=w1691:bool)
            n1651 = local write "Cap Live Image"(w1691) -> ()
            n1652 = case shown="\"ISO 12156\"" w1689 {
              tunnel: ["ASTM D6079" "ISO 12156"] -> w1688
              frame "ASTM D6079", Default {
              }
              frame "ISO 12156" {
              }
            }
            n1653 = case shown="\"5x\", Default" w1701 {
              tunnel: [w1704 w1705] -> w1700
              frame "5x", Default {
                n1654 = local read "5x Gain"() -> (w1704:dbl)
              }
              frame "10x" {
                # "5x"
                n1655 = local read "10x Gain"() -> (w1705:dbl)
              }
            }
            n1656 = local read "Image path"() -> (w1699:path)
            n1657 = local read "FILE 3"() -> (w1692:string)
            n1658 = call "EDGE DETCTION.vi"("GAIN VALUE"=w1700, "Image Path"=w1699) -> ("error out"=w1698:errorcluster, "return value"=w1697:cluster{string, string, dbl, dbl, dbl})  [unwired: 8 in]
            n1659 = Bundle By Name(cluster=T27 {"File Name"="", "Test Method"="", "Operator"="", "Fuel Description"="", "Date and time"=""} ("Main Ref"), "File Name"=w1692, "Test Method"=w1688) -> (w1693:T27)
            n1660 = call "duf file read.vi"("error in (no error)"=w1698, "Main Ref"=w1693) -> ("error out"=w1696:errorcluster, "Main Ref 2"=w1694:T27)  [unwired: 8 in]
            n1661 = call "EDGE DETECTION REPORT.vi"("error in (no error)"=w1696, "return value 2"=w1697, "Main Ref"=w1694) -> ()  [unwired: 8 in, 1 out]
          }
          frame #6 {
            n1662 = property on="Auto Scar Check  2" class="Clust (strict)"("Visible"=FALSE) -> ()  [unwired: 2 in, 2 out]
          }
          frame #7 {
            n1663 = call "CAMERA LIVE FEED FGV.vi"("Enum - Menu"=CAMERA_LIVE_FEED_ENUM."CAMERA MINIMIZE", "error in (no error)"=w1709) -> ()  [unwired: 8 in, 2 out]
            n1664 = local write "Main Dashboard Buttons"(T1."Home" ("Main Dashboard Buttons")) -> ()
            n1665 = local write "Main Tab"(T4."HOME" ("Main Tab")) -> ()
          }
        }
      }
    }
    n1666 = local read "Heater Button"() -> (w1550:bool)
    n1667 = case shown="True" w1552 {
      selector: w1552 -> [_ w1839]
      frame False {
      }
      frame True {
        n1668 = Not(x=w1839) -> (.not. x?=w1837:bool)
        n1669 = local write "Frequency"(w1837) -> ()
        n1670 = local write "Tab Control 2"(T8."Frequency" ("Tab Control 2")) -> ()
      }
    }
    n1671 = case shown="True" w1551 {
      selector: w1551 -> [_ w1836]
      frame False {
      }
      frame True {
        n1672 = Not(x=w1836) -> (.not. x?=w1834:bool)
        n1673 = local write "Air Temp vs Humidity"(w1834) -> ()
        n1674 = local write "Tab Control 2"(T8."Air Temp vs Rh" ("Tab Control 2")) -> ()
      }
    }
    n1675 = case shown="True" w1553 {
      selector: w1553 -> [_ w1842]
      frame False {
      }
      frame True {
        n1676 = Not(x=w1842) -> (.not. x?=w1840:bool)
        n1677 = local write "Sample Temperature"(w1840) -> ()
        n1678 = local write "Tab Control 2"(T8."Sample Temperature" ("Tab Control 2")) -> ()
      }
    }
    n1679 = case shown="\"Custom\"" w1549 {
      frame "ASTM D6079", Default {
        w1815 = "ASTM D6079 TEST CONDITIONS" ("Standard 2")
        n1680 = local write "Standard 2"(w1815) -> ()
        n1681 = local write "Standard"(w1815) -> ()
      }
      frame "ISO 12156" {
        w1816 = "ISO 12156 TEST CONDITIONS" ("Standard 2")
        n1682 = local write "Standard 2"(w1816) -> ()
        n1683 = local write "Standard"(w1816) -> ()
      }
      frame "CEC F-096-A-06" {
        w1817 = "CEC F-096-A-06 TEST CONDITIONS" ("Standard 2")
        n1684 = local write "Standard 2"(w1817) -> ()
        n1685 = local write "Standard"(w1817) -> ()
      }
      frame "Custom" {
        w1818 = "CUSTOM TEST CONDITIONS" ("Standard 2")
        n1686 = local write "Standard 2"(w1818) -> ()
        n1687 = local write "Standard"(w1818) -> ()
      }
    }
    n1688 = case shown="True" w1550 {
      frame False {
        n1689 = local write "Temperature On Command"(TRUE ("Temperature On Command")) -> ()
        n1690 = case shown="True" "Temperature Off Command" {
          selector: "Temperature Off Command" -> [_ w1822]
          frame False {
          }
          frame True {
            n1691 = Not(x=w1822) -> (.not. x?=w1821:bool)
            n1692 = local read "EVENT LOG"() -> (w1825:string)
            n1693 = local write "Temperature Off Command"(w1821) -> ()
            n1694 = call "Event Log.vi"("Content"="Heater Off", "EVENT LOG"=w1825) -> ("EVENT LOG"=w1824:string)  [unwired: 8 in, 1 out]
            n1695 = local write "EVENT LOG"(w1824) -> ()
          }
        }
      }
      frame True {
        n1696 = local write "Temperature Off Command"(TRUE ("Temperature Off Command")) -> ()
        n1697 = case shown="True" "Temperature On Command" {
          selector: "Temperature On Command" -> [_ w1829]
          frame False {
          }
          frame True {
            n1698 = Not(x=w1829) -> (.not. x?=w1828:bool)
            n1699 = local write "Temperature On Command"(w1828) -> ()
            n1700 = disable-structure shown="Enabled" {
              disable-tunnel: "Heater On" -> [w1831 _]
              frame Enabled {
                n1701 = local read "EVENT LOG"() -> (w1832:string)
                n1702 = call "Event Log.vi"("Content"=w1831, "EVENT LOG"=w1832) -> ("EVENT LOG"=w1833:string)  [unwired: 8 in, 1 out]
                n1703 = local write "EVENT LOG"(w1833) -> ()
              }
              frame Disabled {
              }
            }
          }
        }
      }
    }
    n1704 = property on="DEMO" class="Bool (strict)"() -> ("Value"=w1539:bool)  [unwired: 2 in, 2 out]
    n1705 = case shown="False" w1539 {
      frame False {
        n1706 = local read "Main Tab"() -> (w1580:T4)
        n1707 = case shown="\"About\"" w1580 {
          frame "HOME", Default {
            w1581 = T20."Enabled" ("Disabled")
            n1708 = local read "Service Password enable"() -> (w1583:bool)
            n1709 = property on="Imaging" class="Bool (strict)"("DisabledEnum"=w1581) -> ()  [unwired: 2 in, 2 out]
            n1710 = property on="Dashboard" class="Bool (strict)"("DisabledEnum"=w1581) -> ()  [unwired: 2 in, 2 out]
            n1711 = property on="Test Setup" class="Bool (strict)"("DisabledEnum"=w1581) -> ()  [unwired: 2 in, 2 out]
            n1712 = property on="Analysis" class="Bool (strict)"("DisabledEnum"=w1581) -> ()  [unwired: 2 in, 2 out]
            n1713 = property on="Home" class="Bool (strict)"("DisabledEnum"=w1581) -> ()  [unwired: 2 in, 2 out]
            n1714 = property on="Report" class="Bool (strict)"("DisabledEnum"=w1581) -> ()  [unwired: 2 in, 2 out]
            n1715 = property on="Main Dashboard Buttons" class="RadioBtnsControl (strict)"("DisabledEnum"=w1581) -> ()  [unwired: 2 in, 2 out]
            n1716 = property on="Calibration" class="Bool (strict)"("DisabledEnum"=w1581) -> ()  [unwired: 2 in, 2 out]
            n1717 = case shown="True" w1583 {
              tunnel: [T20."Disabled" ("Disabled") T20."Enabled" ("Disabled")] -> w1582
              frame False {
              }
              frame True {
              }
            }
            n1718 = property on="About" class="Bool (strict)"("DisabledEnum"=w1582) -> ()  [unwired: 2 in, 2 out]
          }
          frame "Test Setup" {
            w1588 = T20."Enabled" ("Disabled")
            n1719 = local read "Service Password enable"() -> (w1587:bool)
            n1720 = property on="Dashboard" class="Bool (strict)"("DisabledEnum"=T20."Disabled" ("Disabled")) -> ()  [unwired: 2 in, 2 out]
            n1721 = property on="Imaging" class="Bool (strict)"("DisabledEnum"=w1588) -> ()  [unwired: 2 in, 2 out]
            n1722 = property on="Analysis" class="Bool (strict)"("DisabledEnum"=w1588) -> ()  [unwired: 2 in, 2 out]
            n1723 = property on="Home" class="Bool (strict)"("DisabledEnum"=w1588) -> ()  [unwired: 2 in, 2 out]
            n1724 = property on="Report" class="Bool (strict)"("DisabledEnum"=w1588) -> ()  [unwired: 2 in, 2 out]
            n1725 = property on="Test Setup" class="Bool (strict)"("DisabledEnum"=w1588) -> ()  [unwired: 2 in, 2 out]
            n1726 = case shown="True" w1587 {
              tunnel: [T20."Disabled" ("Disabled") T20."Enabled" ("Disabled")] -> w1586
              frame False {
              }
              frame True {
              }
            }
            n1727 = property on="About" class="Bool (strict)"("DisabledEnum"=w1586) -> ()  [unwired: 2 in, 2 out]
          }
          frame "Adv Scar" {
            w1595 = T20."Enabled" ("Disabled")
            n1728 = property on="Dashboard" class="Bool (strict)"("DisabledEnum"=T20."Disabled" ("Disabled")) -> ()  [unwired: 2 in, 2 out]
            n1729 = property on="Imaging" class="Bool (strict)"("DisabledEnum"=w1595) -> ()  [unwired: 2 in, 2 out]
            n1730 = property on="Analysis" class="Bool (strict)"("DisabledEnum"=w1595) -> ()  [unwired: 2 in, 2 out]
            n1731 = property on="Home" class="Bool (strict)"("DisabledEnum"=w1595) -> ()  [unwired: 2 in, 2 out]
            n1732 = property on="Report" class="Bool (strict)"("DisabledEnum"=w1595) -> ()  [unwired: 2 in, 2 out]
            n1733 = property on="Test Setup" class="Bool (strict)"("DisabledEnum"=w1595) -> ()  [unwired: 2 in, 2 out]
            n1734 = local read "Service Password enable"() -> (w1593:bool)
            n1735 = case shown="True" w1593 {
              tunnel: [T20."Disabled" ("Disabled") T20."Enabled" ("Disabled")] -> w1592
              frame False {
              }
              frame True {
              }
            }
            n1736 = property on="About" class="Bool (strict)"("DisabledEnum"=w1592) -> ()  [unwired: 2 in, 2 out]
          }
          frame "Calibration" {
            w1598 = T20."Enabled" ("Disabled")
            n1737 = property on="Dashboard" class="Bool (strict)"("DisabledEnum"=T20."Disabled" ("Disabled")) -> ()  [unwired: 2 in, 2 out]
            n1738 = property on="Imaging" class="Bool (strict)"("DisabledEnum"=w1598) -> ()  [unwired: 2 in, 2 out]
            n1739 = property on="Analysis" class="Bool (strict)"("DisabledEnum"=w1598) -> ()  [unwired: 2 in, 2 out]
            n1740 = property on="Home" class="Bool (strict)"("DisabledEnum"=w1598) -> ()  [unwired: 2 in, 2 out]
            n1741 = property on="Report" class="Bool (strict)"("DisabledEnum"=w1598) -> ()  [unwired: 2 in, 2 out]
            n1742 = property on="Test Setup" class="Bool (strict)"("DisabledEnum"=w1598) -> ()  [unwired: 2 in, 2 out]
            n1743 = local read "Service Password enable"() -> (w1600:bool)
            n1744 = property on="Calibration" class="Bool (strict)"("DisabledEnum"=w1598) -> ()  [unwired: 2 in, 2 out]
            n1745 = case shown="True" w1600 {
              tunnel: [T20."Disabled" ("Disabled") T20."Enabled" ("Disabled")] -> w1599
              frame False {
              }
              frame True {
              }
            }
            n1746 = property on="About" class="Bool (strict)"("DisabledEnum"=w1599) -> ()  [unwired: 2 in, 2 out]
          }
          frame "Adv Scar Report" {
            w1606 = T20."Enabled" ("Disabled")
            n1747 = property on="Dashboard" class="Bool (strict)"("DisabledEnum"=T20."Disabled" ("Disabled")) -> ()  [unwired: 2 in, 2 out]
            n1748 = property on="Imaging" class="Bool (strict)"("DisabledEnum"=w1606) -> ()  [unwired: 2 in, 2 out]
            n1749 = property on="Analysis" class="Bool (strict)"("DisabledEnum"=w1606) -> ()  [unwired: 2 in, 2 out]
            n1750 = property on="Home" class="Bool (strict)"("DisabledEnum"=w1606) -> ()  [unwired: 2 in, 2 out]
            n1751 = property on="Report" class="Bool (strict)"("DisabledEnum"=w1606) -> ()  [unwired: 2 in, 2 out]
            n1752 = property on="Test Setup" class="Bool (strict)"("DisabledEnum"=w1606) -> ()  [unwired: 2 in, 2 out]
            n1753 = local read "Service Password enable"() -> (w1605:bool)
            n1754 = case shown="True" w1605 {
              tunnel: [T20."Disabled" ("Disabled") T20."Enabled" ("Disabled")] -> w1604
              frame False {
              }
              frame True {
              }
            }
            n1755 = property on="About" class="Bool (strict)"("DisabledEnum"=w1604) -> ()  [unwired: 2 in, 2 out]
          }
          frame "Compare Files" {
            w1612 = T20."Enabled" ("Disabled")
            n1756 = local read "Service Password enable"() -> (w1611:bool)
            n1757 = property on="Dashboard" class="Bool (strict)"("DisabledEnum"=T20."Disabled" ("Disabled")) -> ()  [unwired: 2 in, 2 out]
            n1758 = property on="Imaging" class="Bool (strict)"("DisabledEnum"=w1612) -> ()  [unwired: 2 in, 2 out]
            n1759 = property on="Analysis" class="Bool (strict)"("DisabledEnum"=w1612) -> ()  [unwired: 2 in, 2 out]
            n1760 = property on="Home" class="Bool (strict)"("DisabledEnum"=w1612) -> ()  [unwired: 2 in, 2 out]
            n1761 = property on="Report" class="Bool (strict)"("DisabledEnum"=w1612) -> ()  [unwired: 2 in, 2 out]
            n1762 = property on="Test Setup" class="Bool (strict)"("DisabledEnum"=w1612) -> ()  [unwired: 2 in, 2 out]
            n1763 = case shown="True" w1611 {
              tunnel: [T20."Disabled" ("Disabled") T20."Enabled" ("Disabled")] -> w1610
              frame False {
              }
              frame True {
              }
            }
            n1764 = property on="About" class="Bool (strict)"("DisabledEnum"=w1610) -> ()  [unwired: 2 in, 2 out]
          }
          frame "Acquire" {
            n1765 = local read "Service Password enable"() -> (w1617:bool)
            n1766 = property on="Test Setup" class="Bool (strict)"("DisabledEnum"=T20."Disabled" ("Disabled")) -> ()  [unwired: 2 in, 2 out]
            n1767 = local read "Auto Start Test"() -> (w1619:bool)
            n1768 = local read "RUN"() -> (w1621:bool)
            n1769 = case shown="True" w1617 {
              tunnel: [T20."Disabled" ("Disabled") T20."Enabled" ("Disabled")] -> w1618
              frame False {
              }
              frame True {
              }
            }
            n1770 = Or(x=w1621, y=w1619) -> (x .or. y?=w1620:bool)
            n1771 = case shown="True" w1620 {
              tunnel: [T20."Enabled" ("Disabled") T20."Disabled" ("Disabled")] -> w1616
              frame False {
              }
              frame True {
              }
            }
            n1772 = property on="About" class="Bool (strict)"("DisabledEnum"=w1618) -> ()  [unwired: 2 in, 2 out]
            n1773 = property on="Imaging" class="Bool (strict)"("DisabledEnum"=w1616) -> ()  [unwired: 2 in, 2 out]
            n1774 = property on="Dashboard" class="Bool (strict)"("DisabledEnum"=w1616) -> ()  [unwired: 2 in, 2 out]
            n1775 = property on="Analysis" class="Bool (strict)"("DisabledEnum"=w1616) -> ()  [unwired: 2 in, 2 out]
            n1776 = property on="Home" class="Bool (strict)"("DisabledEnum"=w1616) -> ()  [unwired: 2 in, 2 out]
            n1777 = property on="Report" class="Bool (strict)"("DisabledEnum"=w1616) -> ()  [unwired: 2 in, 2 out]
            n1778 = property on="Calibration" class="Bool (strict)"("DisabledEnum"=w1616) -> ()  [unwired: 2 in, 2 out]
          }
          frame "About" {
            n1779 = local read "FILE"() -> (w1635:string)
            n1780 = local read "TEST FILE NAM,E SAVED"() -> (w1628:bool)
            n1781 = call <vilib>:"Trim Whitespace.vi"("string"=w1635) -> ("trimmed string"=w1634:string)  [unwired: 1 in]
            n1782 = local read "Auto Start Test"() -> (w1638:bool)
            n1783 = String Length(string=w1634) -> (length=w1633:i32)
            n1784 = Greater?(x=w1633, y=1) -> (0:w1630:bool)
            n1785 = And(x=w1630, y=w1628) -> (x .and. y?=w1629:bool)
            n1786 = local read "RUN"() -> (w1640:bool)
            n1787 = case shown="True" w1629 {
              tunnel: [T20."Disabled" ("Disabled") T20."Enabled" ("Disabled")] -> w1631
              frame False {
              }
              frame True {
              }
            }
            n1788 = Or(x=w1640, y=w1638) -> (x .or. y?=w1639:bool)
            n1789 = property on="About" class="Bool (strict)"("DisabledEnum"=T20."Enabled" ("Disabled")) -> ()  [unwired: 2 in, 2 out]
            n1790 = case shown="False" w1639 {
              tunnel: [T20."Enabled" ("Disabled") T20."Disabled" ("Disabled")] -> w1637
              frame False {
              }
              frame True {
              }
            }
            n1791 = property on="Dashboard" class="Bool (strict)"("DisabledEnum"=w1631) -> ()  [unwired: 2 in, 2 out]
            n1792 = property on="Test Setup" class="Bool (strict)"("DisabledEnum"=T20."Disabled" ("Disabled")) -> ()  [unwired: 2 in, 2 out]
            n1793 = property on="Imaging" class="Bool (strict)"("DisabledEnum"=w1637) -> ()  [unwired: 2 in, 2 out]
            n1794 = property on="Analysis" class="Bool (strict)"("DisabledEnum"=w1637) -> ()  [unwired: 2 in, 2 out]
            n1795 = property on="Home" class="Bool (strict)"("DisabledEnum"=w1637) -> ()  [unwired: 2 in, 2 out]
            n1796 = property on="Report" class="Bool (strict)"("DisabledEnum"=w1637) -> ()  [unwired: 2 in, 2 out]
          }
        }
      }
      frame True {
      }
    }
    n1797 = local read "Quit"() -> (w1565:bool)
